vi "SMO Name - constant.vi"(8 "error in (no error)":errorcluster, 11 "instrument.PPMS2 in":refnum<class "instrument.PPMS.lvclass">) -> (0 "error out":errorcluster, 2 "SMO Name":string, 3 "instrument.PPMS2 out":refnum<class "instrument.PPMS.lvclass">)   [LabVIEW 2016, in "instrument.PPMS.lvclass"]
uses:
  instrument.PPMS.lvclass
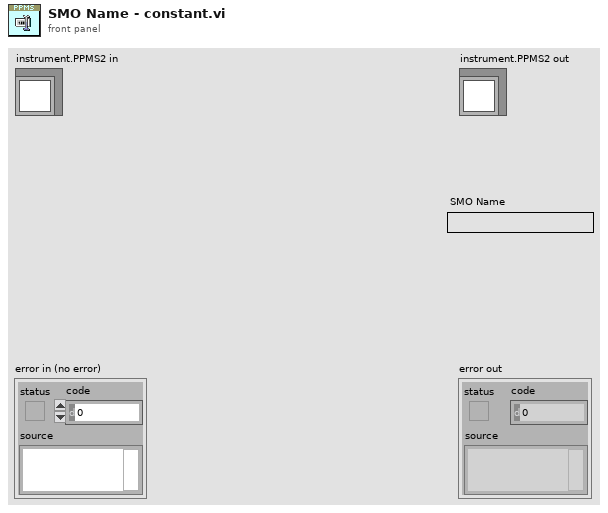
[diagram p1: front panel]
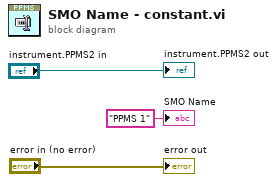
[diagram p0: block diagram]
diagram:
  "error out" <- "error in (no error)"
  "instrument.PPMS2 out" <- "instrument.PPMS2 in"
  "SMO Name" <- "PPMS 1" ("SMO Name")
